vi "XY Sample Stage History Points Holder.vi"(2 "Actions":T1=enum."Read", 7 "(x, y) Points":dbl[](array[numeric]), 13 "Zero Position (x, y)":dbl[](array[numeric])) -> (8 "History Points":cluster{dbl[], dbl[]})   [LabVIEW 2016]
uses:
  XY Sample Stage Controls/XY Sample Stage History Actions.ctl
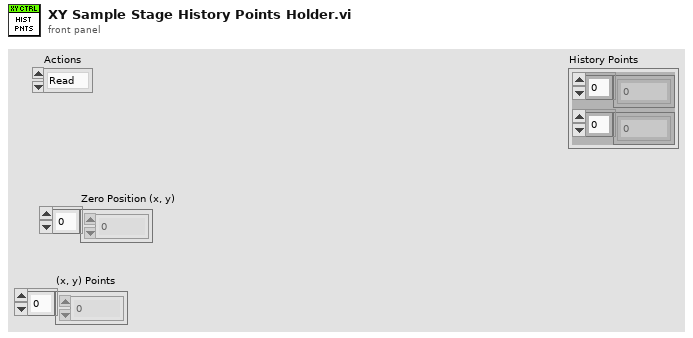
[diagram p1: front panel]
types:
  T1 = typedef "XY Sample Stage History Actions.ctl" = enum16{"Reset", "Write", "Read", "Set Zero"}
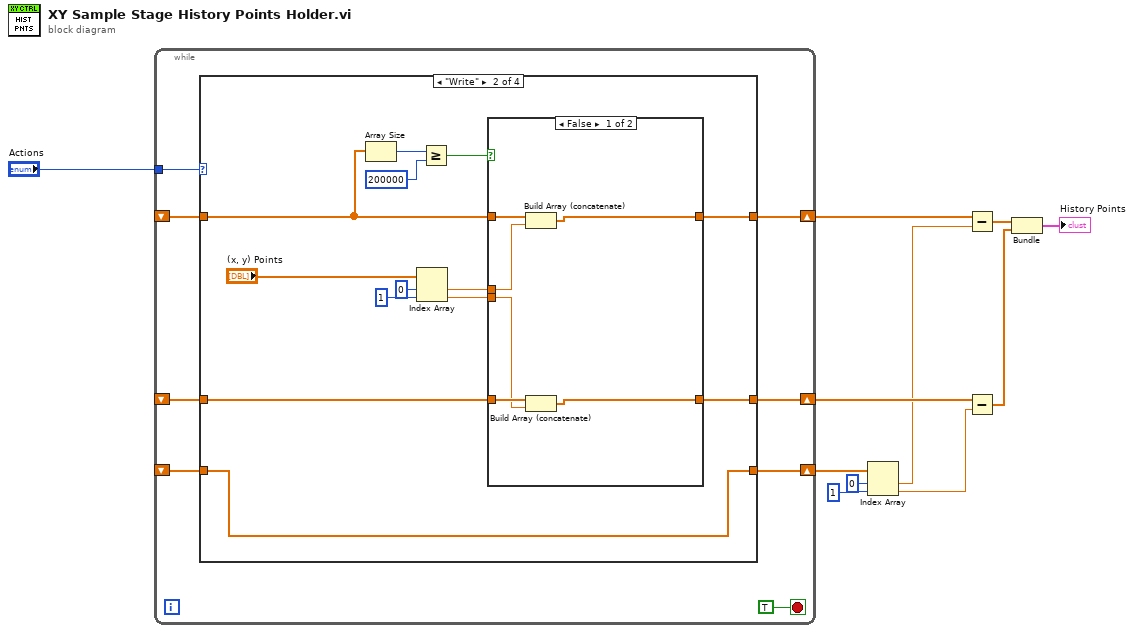
[diagram p0: block diagram]
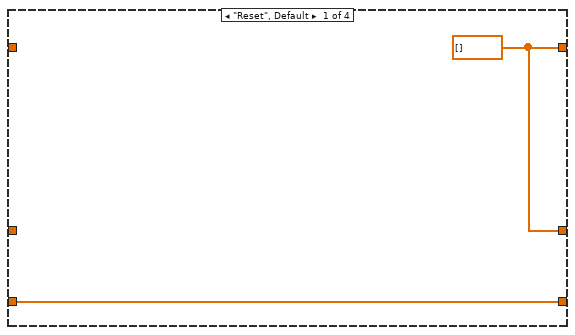
[diagram p2: hidden frame]
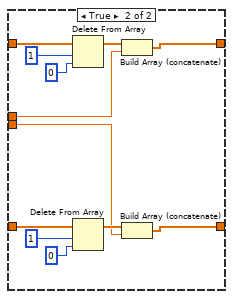
[diagram p3: hidden frame]
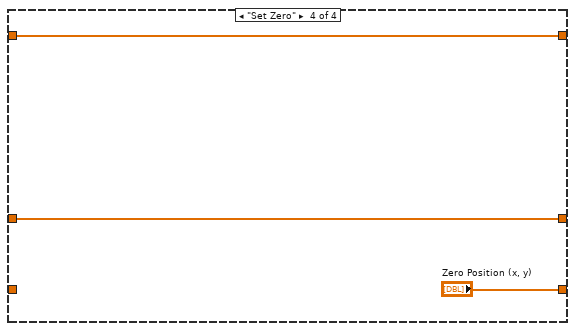
[diagram p5: hidden frame]
diagram:
  n1 = while {
    shift-right: [w17] -> w5
    shift-left: _ -> [w15]
    shift-right: [w16] -> w6
    shift-left: _ -> [w14]
    tunnel: "Actions" -> [w18]
    shift-right: [w13] -> w9
    shift-left: _ -> [w12]
    stop <- TRUE stop-if-true
    n2 = case shown="\"Write\"" w18 {
      tunnel: [w21 w25 w55 w58] -> w17
      tunnel: [w21 w24 w54 w57] -> w16
      tunnel: w15 -> [_ w29 w55 w58]
      tunnel: w14 -> [_ w28 w54 w57]
      tunnel: [w20 w23 w53 "Zero Position (x, y)"] -> w13
      tunnel: w12 -> [w20 w23 w53 _]
      frame "Reset", Default {
        w21 = dbl[] []
      }
      frame "Write" {
        n3 = Array Size(array=w29) -> (size(s)=w34:i32)
        n4 = Index Array(array="(x, y) Points", index #1=0 ("index"), index #2=1 ("index")) -> (element #1=w27:dbl, element #2=w26:dbl)
        n5 = Greater Or Equal?(x=w34, y=200000) -> (x >= y?=w32:bool)
        n6 = case shown="False" w32 {
          tunnel: w29 -> [w40 w52]
          tunnel: w28 -> [w39 w47]
          tunnel: w27 -> [w37 w44]
          tunnel: w26 -> [w38 w43]
          tunnel: [w36 w42] -> w25
          tunnel: [w35 w41] -> w24
          frame False {
            n7 = Build Array (concatenate)(w40, w37) -> (w36:dbl[])
            n8 = Build Array (concatenate)(w39, w38) -> (w35:dbl[])
          }
          frame True {
            n9 = Delete From Array(array=w52, length=1, index=0 ("length")) -> (array with subset deleted=w46:dbl[])  [unwired: 1 out]
            n10 = Delete From Array(array=w47, length=1, index=0 ("length")) -> (array with subset deleted=w45:dbl[])  [unwired: 1 out]
            n11 = Build Array (concatenate)(w46, w44) -> (w42:dbl[])
            n12 = Build Array (concatenate)(w45, w43) -> (w41:dbl[])
          }
        }
      }
      frame "Read" {
      }
      frame "Set Zero" {
      }
    }
  }
  n13 = Index Array(array=w9, index #1=0 ("index"), index #2=1 ("index")) -> (element #1=w2:dbl, element #2=w1:dbl)
  n14 = Subtract(x=w5, y=w2) -> (x-y=w4:dbl[])
  n15 = Subtract(x=w6, y=w1) -> (x-y=w3:dbl[])
  n16 = Bundle(w4, w3) -> (→"History Points":cluster{dbl[], dbl[]})  [unwired: 1 in]
